vi "CSGaussmeter.constructor.vi"(0 "name":string, 2 "data in":string, 5 "error in (no error)":errorcluster) -> (14 "i ref out":refnum<vi>, 16 "data out":string, 19 "error out":errorcluster)   [LabVIEW 2014, in "CSGaussmeter.lvlib"]
doc: "This is the constructor of a class.\n\nLicense Agreement for this software:\n\nCopyright (C)\nGesellschaft für Schwerionenforschung, GSI\nPlanckstr. 1\n64291 Darmstadt\nGermany\n\nContact: D.Beck@gsi.de \n\nThis program is free software; you can redistribute it and/or modify it under the terms of the \nGNU General Public License as published by the Free Software Foundation; either version 2 of \nthe license, or (at your option) any later version.\n\nThis program is distributed in the hope that it will be useful, but WITHOUT ANY WARRANTY; \nwithout even the implied warranty of MERCHANTABILITY or FITNESS FOR A PARTICULAR PURPOSE. See the GNU General License for more details (http://www.gnu.org).\n\nGesellschaft für Schwerionenforschung, GSI\nPlanckstr. 1, 64291 Darmstadt, Germany\nFor all questions and ideas contact: M.Richter@gsi.de, H.Brand@gsi.de or D.Beck@gsi.de.\nLast update: 16-JUN-2004"
uses:
  CSGaussmeter.lvlib
  CSGaussmeter.i attribute.ctl
  instr.lib/FH_55/TypeDef/Unit.ctl
  instr.lib/FH_55/TypeDef/Temp_Unit.ctl
  instr.lib/FH_55/TypeDef/Max.ctl
  instr.lib/FH_55/TypeDef/Range.ctl
  instr.lib/FH_55/TypeDef/Unit2.ctl
  instr.lib/FH_55/TypeDef/Display.ctl
  instr.lib/FH_55/TypeDef/Value_String.ctl
  CS_Core/CSApplicationBaseClasses/DeviceBase/DeviceBase.lvlib
  CS_Core/CSSystem/CSSystemLib/CSSystemLib.lvlib
  CS_Core/BaseProcess/BaseProcess.lvlib
  instr.lib/FH_55/FH 55.lvlib
panel:
  in  "CLASS.i attribute":T1 {"setValues"."Set_Rel"."Numeric" format="%#_4f"; "setValues"."Set_upper"."Numeric" format="%#_4f"; "setValues"."Set_lower"."Numeric" format="%#_4f"; "actValues"."Set_Rel"."Numeric" format="%#_4f"; "actValues"."Set_upper"."Numeric" format="%#_4f"; "actValues"."Set_lower"."Numeric" format="%#_4f"}
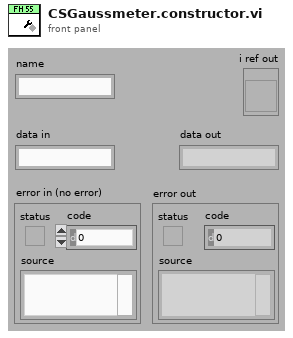
[diagram p1: front panel]
types:
  T1 = typedef "CSGaussmeter.lvlib/CSGaussmeter.i attribute.ctl" = cluster{"Name":string, "VISA Resource Name":refnum<visa-resource-name>, "actValues":cluster{" Limit":bool, "Unit ":T2, "Temp_Unit":T3, "Max":T4, " Filter":bool, " Peak":bool, " Auto_Range":bool, "Range":T5, " Rel":bool, " CTemp":bool, " CField":bool, "AC_DC ":bool, "Set_lower":cluster{"Numeric":dbl, "Cancel Button":bool, "Unit":T6}, "Set_upper":cluster{"Numeric":dbl, "Cancel Button":bool, "Unit":T6}, "Set_Rel":cluster{"Numeric":dbl, "Cancel Button":bool, "Unit":T6}, "Zero":bool, " Local":bool, "Reset":bool, " Init":bool}, "FH 55 Gauss-/Teslameter":T7, "MAX_Value":T8, "MIN_Value":T8, "Rel_Value":T8, "Array ":string[], "LIMU":dbl, " LIML":dbl, "Messwerte 2":string, "Messwerte ":cluster{"Numeric":i32, "OK Button":bool}, "serviceID":cluster{"Current ID":i32, "Unit ID":i32, "Temp ID":i32, "Name ID \n":i32, "Visa ID ":i32}, "setValues ":cluster{" Limit":bool, "Unit ":T2, "Temp_Unit":T3, "Max":T4, " Filter":bool, " Peak":bool, " Auto_Range":bool, "Range":T5, " Rel":bool, " CTemp":bool, " CField":bool, "AC_DC ":bool, "Set_lower":cluster{"Numeric":dbl, "Cancel Button":bool, "Unit":T6}, "Set_upper":cluster{"Numeric":dbl, "Cancel Button":bool, "Unit":T6}, "Set_Rel":cluster{"Numeric":dbl, "Cancel Button":bool, "Unit":T6}, "Zero":bool, " Local":bool, "Reset":bool, " Init":bool}}
  T2 = typedef "FH 55.lvlib/Unit.ctl" = enum16{"T", "G", "A/m"}
  T3 = typedef "FH 55.lvlib/Temp_Unit.ctl" = enum16{"Temp off", "Celsius", "Fahrenheit"}
  T4 = typedef "FH 55.lvlib/Max.ctl" = enum16{"MAX off", "Show MAX", "MAX/MIN"}
  T5 = typedef "FH 55.lvlib/Range.ctl" = enum16{"1", "2", "3", "4", "5", "6", "7"}
  T6 = typedef "FH 55.lvlib/Unit2.ctl" = enum16{"mT", "G", "kA/m"}
  T7 = typedef "FH 55.lvlib/Display.ctl" = cluster{"current value":string, "Limit":string, "Remote":string, "function ":string, "Cluster":cluster{"AC/DC":string, "Auto":string, "Filter":string, "Range":string, "Rel":string, "Peak":string}}
  T8 = typedef "FH 55.lvlib/Value_String.ctl" = cluster{"Numeric":dbl, "String":string}
  T9 = enum16{"SetAttribute", "GetAttribute", "CreateAttribute", "DestroyAttribute", "DestroyAllAtributes"}
  T10 = typedef "BaseProcess.lvlib/BaseProcess.i attribute.ctl" = cluster{"EventStatus":string, "EventError":i32, "PresetEvtWatchD":i32, "PresetPdcWatchD":i32, "EventTimeout":i32, "PeriodicInterval":i32, "Interface":string[], "Address":string[], "Special":string[], "PeriodicError":i32, "PeriodicStatus":string, "SuperProc":string, "Descriptors":T11[], "CaseRef":refnum<vi>, "PdcRef":refnum<vi>, "Thread Ref":refnum<vi>, "eventErrorID":i32, "eventStatusID":i32, "periodicErrorID":i32, "periodicStatusID":i32, "pdcCtrID":i32}
  T11 = typedef "BaseProcess.lvlib/BaseProcess.descriptor definition.ctl" = cluster{"selector":string, "descriptor":T12}
  T12 = typedef "BaseProcess.lvlib/BaseProcess.descriptor string definition.ctl" = string
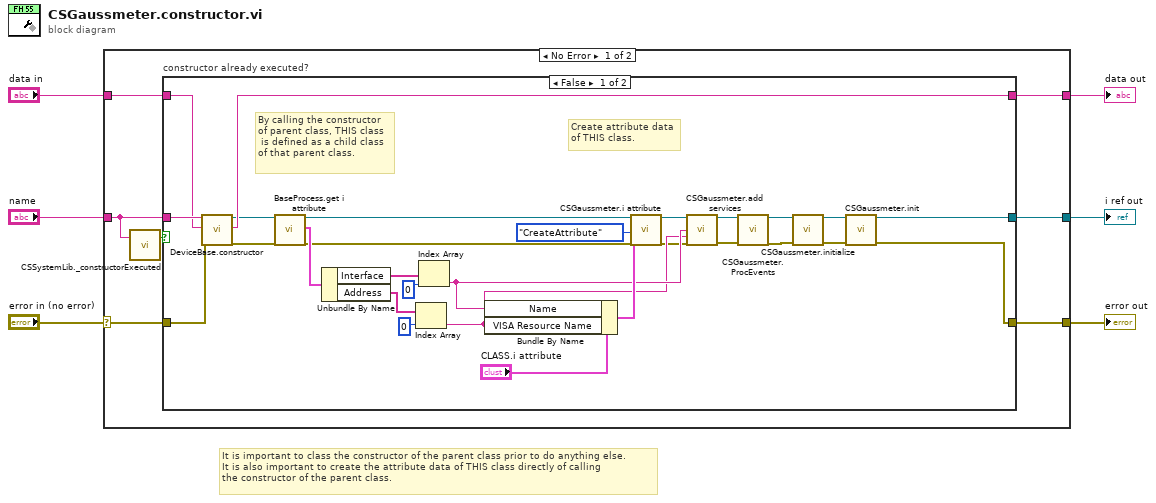
[diagram p0: block diagram]
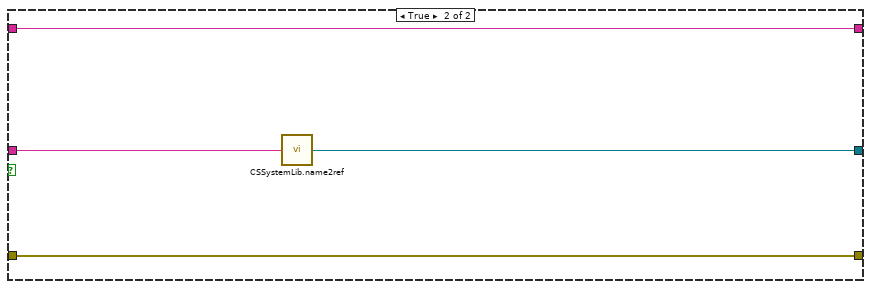
[diagram p2: hidden frame]
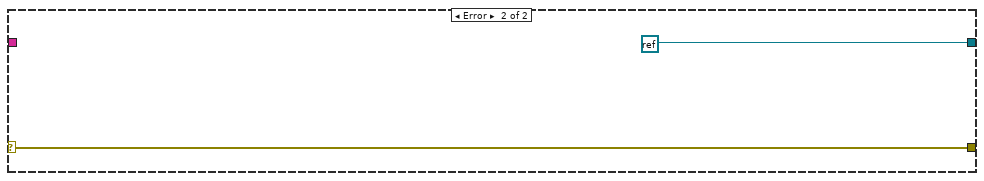
[diagram p3: hidden frame]
diagram:
  # "It is important to class the constructor of the parent class prior to do anything else.\nIt is also important to create the attribute data of THIS class directly of calling\nthe constructor of the parent class."
  n1 = case shown="No Error" "error in (no error)" {
    selector: "error in (no error)" -> [w11 w46]
    tunnel: "name" -> [w10 _]
    tunnel: [w13 refnum<k0> refnum ("Not a Refnum Constant")] -> w5
    tunnel: [w12 w46] -> w4
    tunnel: "data in" -> [w8 _]
    tunnel: [w7 _] -> w1
    frame No Error {
      n2 = call "CSSystemLib._constructorExecuted.vi"("name"=w10) -> ("constructor executed?"=w9:bool)  [unwired: 18 in]
      n3 = case "constructor already executed?" shown="False" w9 {
        tunnel: w10 -> [w40 w45]
        tunnel: [w25 w44] -> w13
        tunnel: [w14 w43] -> w12
        tunnel: w11 -> [w39 w43]
        tunnel: w8 -> [w38 w42]
        tunnel: [w37 w42] -> w7
        frame False {
          # "Create attribute data\nof THIS class."
          # "By calling the constructor\nof parent class, THIS class\n is defined as a child class\nof that parent class."
          n4 = call "DeviceBase.constructor.vi"("name"=w40, "data in"=w38, "error in (no error)"=w39) -> ("i ref out"=w31:refnum<vi>, "data out"=w37:string, "error out"=w30:errorcluster)  [unwired: 14 in]
          n5 = call "BaseProcess.get i attribute.vi"("i ref in"=w31, "error in (no error)"=w30) -> ("i ref out"=w27:refnum<vi>, "i attribute"=w32:T10, "error out"=w28:errorcluster)  [unwired: 15 in]
          n6 = Unbundle By Name(w32) -> ("Interface"=w36:string[], "Address"=w34:string[])
          n7 = Index Array(array=w34, index=0) -> (element=w19:string)
          n8 = Index Array(array=w36, index=0) -> (element=w20:string)
          n9 = Bundle By Name(cluster="CLASS.i attribute", "Name"=w20, "VISA Resource Name"=w19) -> (w26:T1)
          n10 = call "CSGaussmeter.i attribute.vi"("VI Refnum"=w27, "CLASS.i attribute"=w26, "Action"=T9."CreateAttribute", "error in (no error)"=w28) -> ("VI Refnum out"=w22:refnum<vi>, "error out"=w18:errorcluster)  [unwired: 13 in, 1 out]
          n11 = call "CSGaussmeter.add services.vi"("i ref in"=w22, "Name"=w20, "VISA Resource Name"=w19, "error in (no error)"=w18) -> ("i ref out"=w21:refnum<vi>, "error out"=w17:errorcluster)  [unwired: 9 in, 1 out]
          n12 = call "CSGaussmeter.ProcEvents.vi"("i ref in"=w21, "error in (no error)"=w17) -> ("i ref out"=w24:refnum<vi>, "error out"=w23:errorcluster)  [unwired: 16 in]
          n13 = call "CSGaussmeter.initialize.vi"("i ref in"=w24, "error in"=w23) -> ("i ref out"=w16:refnum<vi>, "error out"=w15:errorcluster)  [unwired: 12 in]
          n14 = call "CSGaussmeter.init.vi"("i ref in"=w16, "error in"=w15) -> ("i ref out"=w25:refnum<vi>, "error out"=w14:errorcluster)  [unwired: 12 in]
        }
        frame True {
          n15 = call "CSSystemLib.name2ref.vi"("name"=w45) -> ("obj refnum"=w44:refnum<vi>)
        }
      }
    }
    frame Error {
    }
  }
  "i ref out" <- w5
  "error out" <- w4
  "data out" <- w1
